vi "STA - Wave V0 Host.vi"() -> ()   [LabVIEW 2015]
doc: "The continuous acquisition mode tells the FPGA to acquire points indefinitely until a stop command is issued or until an error is encountered (FIFO overflow, module underflow, and so on). \n\nIn this acquisition mode, explicitly call the appropriate rwfm_ConfigTiming VI and set the host application's data buffer to be many times larger than the read size. The examples use a 10X size by default. If the host application's data buffer fills, then the FPGA experiences a FIFO overflow causing the acquisition to stop."
uses:
  <vilib>/NI/cRIO Wfm/ChannelConfig.ctl
  <vilib>/FPGAPlugInAG/cRIO-9112/niLvFpga_Open_cRIO-9112.vi
  <vilib>/rvi/interface/common/dynamic/niFpgaDynamicAddResources.vi
  <vilib>/NI/cRIO Wfm/AcqRead(Wfm).vi
  <vilib>/FPGAPlugInAG/Dynamic/niLvFpga_Close_Dynamic.vi
  <vilib>/rvi/interface/nirviOpenFPGA/nirviOpenFPGA.xnode
  FPGA Bitfiles/STA-WaveformV0_FPGATarget2_[FPGA]DeltaSigMa_17CDL+fh61Q.lvbitx
  FPGA/[FPGA] DeltaSig Main.vi
  <vilib>/rvi/interface/nirviCloseFPGA/nirviCloseFPGA.xnode
  <vilib>/NI/cRIO Wfm/cRIO Wfm.lvlib
  FPGA Bitfiles/SARAcqMain_9074.lvbitx
  C:/Program Files (x86)/National Instruments/LabVIEW 2015/ProjectTemplates/Source/cRIOWfm/FPGA/[FPGA] SAR Acq Main.vi
panel:
  out "file path":path
  out "error out 2":errorcluster
  in  "error in (no error)":errorcluster
  out "error out":errorcluster
  in  "Sample Rate":u32=51200
  in  "stop":bool
  out "Waveform Graph":waveform(sgl)[](graph)
  in  "Channel Info":T1=[{"Channel Name"="Mod1/ai0", "Sensitivity mV_EU"=1000.0, "EU"="V", "dB Ref EU"=1.0}, {"Channel Name"="Mod1/ai1", "Sensitivity mV_EU"=1000.0, "EU"="V", "dB Ref EU"=1.0}, {"Channel Name"="Mod1/ai2", "Sensitivity mV_EU"=1000.0, "EU"="V", "dB Ref EU"=1.0}, {"Channel Name"="Mod1/ai3", "Sensitivity mV_EU"=1000.0, "EU"="V", "dB Ref EU"=1.0}] caption="Channel Name      Scale [mV/EU]        EU           dB Ref [EU]" {"dB Ref EU" format="%#.2p"; "Sensitivity mV_EU" format="%.2f"}
  in  "Samps per Chan":i32=25600 caption="Samples per Channel"
  out "Buffer Backlog":dbl caption="RT Buffer Backlog [%]" format="%#.2g"
  # "Sampling Info"
  # "Channel Info"
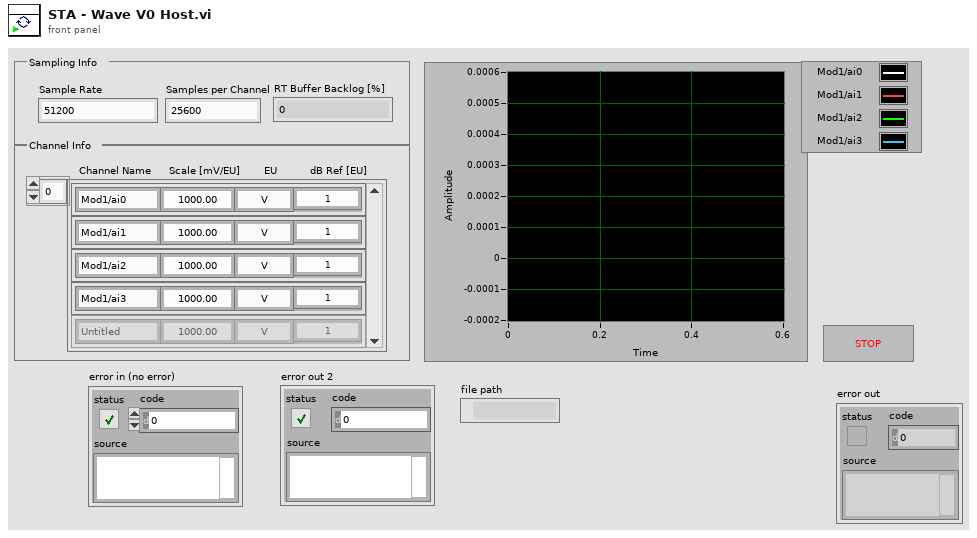
[diagram p1: front panel]
types:
  T1 = typedef "cRIO Wfm.lvlib/ChannelConfig.ctl" = cluster{"Channel Name":string, "Sensitivity mV_EU":dbl, "EU":string, "dB Ref EU":dbl}[]
  T2 = enum16{"open", "open or create", "create or replace", "create", "open (read-only)"}
  T3 = typedef "cRIO Wfm.lvlib/SamplingInfo.ctl" = cluster{"Number of Channels":i32, "Actual Samp Rate":dbl, "Chan Name Array":string[], "EU Chan Array":string[], "dB Ref Chan Array":dbl[]}
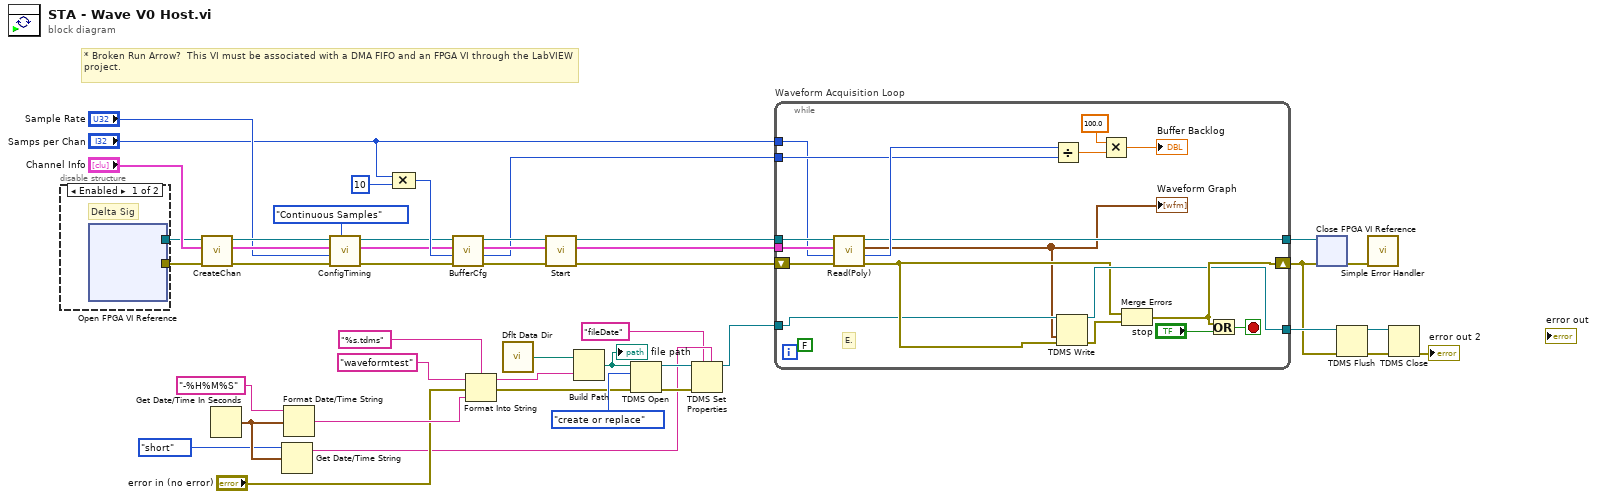
[diagram p0: block diagram]
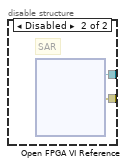
[diagram p2: hidden frame]
diagram:
  # "* Broken Run Arrow?  This VI must be associated with a DMA FIFO and an FPGA VI through the LabVIEW project."
  n1 = disable-structure shown="Enabled" {
    disable-tunnel: [w47 w49] -> w24
    disable-tunnel: [w46 w48] -> w23
    frame Enabled {
      # "Delta Sig"
      n2 = xnode "Open FPGA VI Reference"() -> ("FPGA VI Reference Out"=w47:refnum<k20>, "error out"=w46:errorcluster)  [unwired: 2 in]
    }
    frame Disabled {
      # "SAR"
      n3 = xnode "Open FPGA VI Reference"() -> ("FPGA VI Reference Out"=w49:refnum<k20>, "error out"=w48:errorcluster)  [unwired: 2 in]
    }
  }
  n4 = call <vilib>:"CreateChan.vi"("error in"=w23, "Channel Info"="Channel Info", "Dynamic FPGA Ref"=w24) -> ("error out"=w28:errorcluster, "Sampling Info"=w32:T3, "Dynamic FPGA Ref Out"=w33:refnum<k20>)  [unwired: 1 in, 5 out]
  n5 = Get Date/Time In Seconds() -> (seconds since 1Jan1904=w12:timestamp)
  n6 = Get Date/Time String(date format (0)=enum16{"short", "long", "abbreviated"}."short", seconds (now)=w12) -> (date string=w11:string)  [unwired: 1 in, 1 out]
  n7 = Format Date/Time String(time format string (%c)="-%H%M%S", seconds (now)=w12) -> (date/time string=w16:string)  [unwired: 1 in]
  n8 = call <vilib>:"ConfigTiming.vi"("Sample Mode"=enum16{"Finite Samples", "Continuous Samples"}."Continuous Samples", "error in"=w28, "Sample Rate"="Sample Rate", "Sampling Info In"=w32, "Dynamic FPGA Ref"=w33) -> ("error out"=w29:errorcluster, "Sampling Info Out"=w30:T3, "Dynamic FPGA Ref Out"=w31:refnum<k20>)  [unwired: 3 in, 1 out]
  n9 = Compound Arithmetic op=MULTIPLY("Samps per Chan", 10 ("value")) -> (w38:i32)
  n10 = call <vilib>:"BufferCfg.vi"("error in"=w29, "Buffer Size [Samps per Chan]"=w38, "Sampling Info In"=w30, "Dynamic FPGA Ref"=w31) -> ("error out"=w39:errorcluster, "Buffer Size [Total Samples]"=w35:u32, "Sampling Info Out"=w37:T3, "Dynamic FPGA Ref Out"=w40:refnum<k20>)  [unwired: 4 out]
  n11 = Format Into String(format string="%s.tdms", initial string="waveformtest", error in="error in (no error)", w16) -> (resulting string=w20:string, error out=w14:errorcluster)
  n12 = call <vilib>:"Dflt Data Dir.vi"() -> ("App:Default Data Directory"=w8:path)
  n13 = call <vilib>:"Start.vi"("error in"=w39, "Sampling Info In"=w37, "Dynamic FPGA Ref"=w40) -> ("error out"=w44:errorcluster, "Sampling Info Out"=w36:T3, "Dynamic FPGA Ref Out"=w45:refnum<k20>)  [unwired: 6 out]
  n14 = Build Path(base path=w8, name or relative path=w20) -> (appended path=w1:path)
  "file path" <- w1
  n15 = TDMS Open(8:w14, 10:T2."create or replace" ("operation (0:open)"), 11:w1) -> (0:w22:errorcluster, 3:w13:refnum<k34>)  [unwired: 4 in]
  n16 = TDMS Set Properties(5:w11, 7:"fileDate" ("property names"), 8:w22, 11:w13) -> (3:w7:refnum<k34>)  [unwired: 2 in, 3 out]
  n17 = while "Waveform Acquisition Loop" {
    tunnel: w45 -> [w60]
    tunnel: [w56] -> w43
    tunnel: w36 -> [w66]
    tunnel: w35 -> [w64]
    tunnel: "Samps per Chan" -> [w57]
    shift-right: [w55] -> w5
    shift-left: w44 -> [w67]
    tunnel: w7 -> [w51]
    tunnel: [w53] -> w6
    stop <- w59 stop-if-true
    (unwired) FALSE ("append to file? (new file:F)")
    # "E."
    n18 = call-poly <vilib>:"Read(Poly).vi"("error in"=w67, "Samps Read per Chan"=w57, "Sampling Info"=w66, "Dynamic FPGA Ref"=w60) -> ("error out"=w52:errorcluster, "Samples Remaining"=w65:u32, "Wfm Data"=w50:waveform(sgl)[], "Dynamic FPGA Ref Out"=w56:refnum<k20>)  [unwired: 2 in, 2 out]
    "Waveform Graph" <- w50
    n19 = Divide(x=w65, y=w64) -> (x/y=w63:dbl)
    n20 = TDMS Write(0:w51, 9:w50, 11:w52) -> (4:w53:refnum<k34>, 15:w54:errorcluster)  [unwired: 3 in, 2 out]
    n21 = Multiply(x=100.0, y=w63) -> (x*y=→"Buffer Backlog":dbl)
    n22 = Merge Errors(w52, w54) -> (w55:errorcluster)
    n23 = Or(x=w55, y="stop") -> (x .or. y?=w59:bool)
  }
  n24 = xnode "Close FPGA VI Reference"("FPGA VI Reference In"=w43, "error in"=w5) -> ("error out"=w41:errorcluster)
  n25 = TDMS Flush(4:w5, 7:w6) -> (0:w3:errorcluster, 3:w4:refnum<k34>)
  n26 = call <vilib>:"Simple Error Handler.vi"("error in (no error)"=w41) -> ()  [unwired: 1 in, 8 out]
  n27 = TDMS Close(8:w3, 11:w4) -> (0:→"error out 2":errorcluster)  [unwired: 1 out]
